vi "Enqueue Error.vi"(9 "error to process":errorcluster, 10 "Error Type (Non-Critical)":T1, 11 "Block information (which loop the error happens)":string) -> (0 "error out":errorcluster)   [LabVIEW 2018, in "Message Queue.lvlib"]
uses:
  Message Queue.lvlib
  Error Type.ctl
  error queue name (constant).ctl
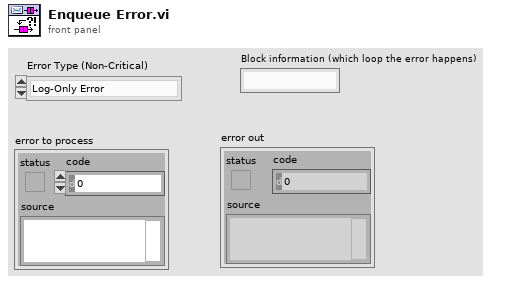
[diagram p1: front panel]
types:
  T1 = typedef "Message Queue.lvlib/Error Type.ctl" = enum16{"Log-Only Error", "Non-Critical Error", "Critical Error"}
  T2 = typedef "Message Queue.lvlib/error queue name (constant).ctl" = string
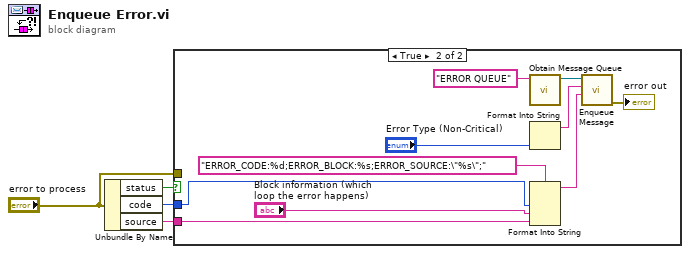
[diagram p0: block diagram]
diagram:
  n1 = Unbundle By Name("error to process") -> ("status"=w3:bool, "code"=w2:i32, "source"=w1:string)
  n2 = case shown="True" w3 {
    tunnel: "error to process" -> [_ _]
    tunnel: w2 -> [_ w8]
    tunnel: w1 -> [_ w5]
    frame False {
    }
    frame True {
      n3 = call "Obtain Message Queue.vi"("name (unnamed)"=T2 "ERROR QUEUE") -> ("Message Queue"=w11:refnum<queue>)  [unwired: 8 in, 2 out]
      n4 = Format Into String("Error Type (Non-Critical)") -> (resulting string=w13:string)  [unwired: 3 in, 1 out]
      n5 = Format Into String(format string="ERROR_CODE:%d;ERROR_BLOCK:%s;ERROR_SOURCE:\"%s\";", w8, "Block information (which loop the error happens)", w5) -> (resulting string=w7:string)  [unwired: 2 in, 1 out]
      n6 = call "Enqueue Message.vi"("Message Data"=w7, "Message"=w13, "Message Queue"=w11) -> ("error out"=→"error out":errorcluster)  [unwired: 7 in, 1 out]
    }
  }
